vi "MGCC_Commun_ConvertDigitalOutput (SubVI).vi"(11 "Reset?":T1[](array[typedef]) {"Control" items=["Nul"=0, "Pulse On"=1, "Pulse Off"=2, "Latch On"=3, "Latch Off"=4, "Close"=65, "Trip"=129]}) -> (3 "Array":bool[](array[boolean]))   [LabVIEW 2016]
uses:
  <vilib>/DNP3/DNP3_Common/crob.ctl
  <vilib>/DNP3/DNP3_Common/crob_ctrl.ctl
  <vilib>/DNP3/DNP3_Common.lvlib
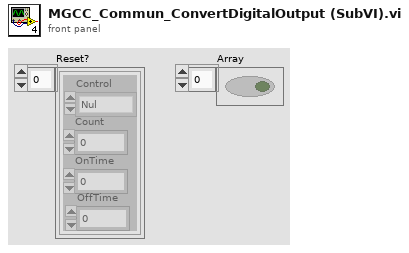
[diagram p1: front panel]
types:
  T1 = typedef "DNP3_Common.lvlib/crob.ctl" = cluster{"OnTime":u32, "Count":u8, "OffTime":u32, "Control":T2}
  T2 = typedef "DNP3_Common.lvlib/crob_ctrl.ctl" = u8
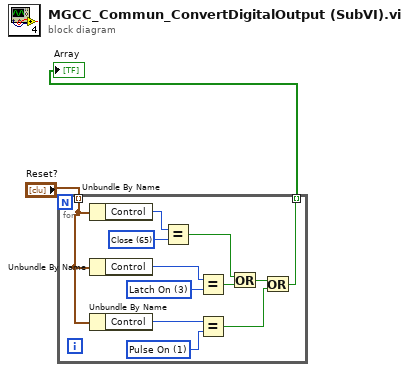
[diagram p0: block diagram]
diagram:
  n1 = for {
    tunnel: "Reset?" -> [w4] mode=indexing
    tunnel: [w3] -> w2 mode=indexing
    w8 = T2 1 items=["Nul"=0, "Pulse On"=1, "Pulse Off"=2, "Latch On"=3, "Latch Off"=4, "Close"=65, "Trip"=129] ("x")
    w12 = T2 65 items=["Nul"=0, "Pulse On"=1, "Pulse Off"=2, "Latch On"=3, "Latch Off"=4, "Close"=65, "Trip"=129] ("x")
    w13 = T2 3 items=["Nul"=0, "Pulse On"=1, "Pulse Off"=2, "Latch On"=3, "Latch Off"=4, "Close"=65, "Trip"=129] ("x")
    n2 = Unbundle By Name(w4) -> ("Control"=w11:T2)
    n3 = Unbundle By Name(w4) -> ("Control"=w14:T2)
    n4 = Unbundle By Name(w4) -> ("Control"=w7:T2)
    n5 = Equal?(x=w11, y=w12) -> (x = y?=w9:bool)
    n6 = Equal?(x=w14, y=w13) -> (x = y?=w10:bool)
    n7 = Equal?(x=w7, y=w8) -> (x = y?=w6:bool)
    n8 = Or(x=w9, y=w10) -> (x .or. y?=w5:bool)
    n9 = Or(x=w5, y=w6) -> (x .or. y?=w3:bool)
  }
  "Array" <- w2
